vi "alinha-com-parede.vi"(4 "NXT/EV3":T1) -> (1 "NXT/EV3 2":T1)   [LabVIEW 2016]
uses:
  <vilib>/NXT/Subs/LVHSConnector.ctl
  <vilib>/NXT/LegoClasses/BrickReference/BrickReference.lvclass
  <vilib>/NXT/Block Support/NXT_InputPort.ctl
  <vilib>/NXT/Block Support/NXT_OutputPort.ctl
  <vilib>/NXT/Dual Mode Library/Sensors/Touch_Pressed.vi
  <vilib>/NXT/NXTIO Xnodes/NXTIONodeSubVIs/NXTMoveMotors.vi
  <vilib>/NXT/NXTIO Xnodes/AddressXNode/NXTIOAddress.xnode
  <vilib>/NXT/NXTIO Xnodes/NXTIOXNode/NXTIO.xnode
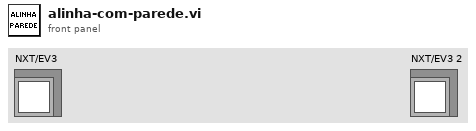
[diagram p1: front panel]
types:
  T1 = typedef "LVHSConnector.ctl" = refnum<class "BrickReference.lvclass">
  T2 = typedef "NXT_OutputPort.ctl" = u8
  T3 = typedef "NXT_InputPort.ctl" = u32
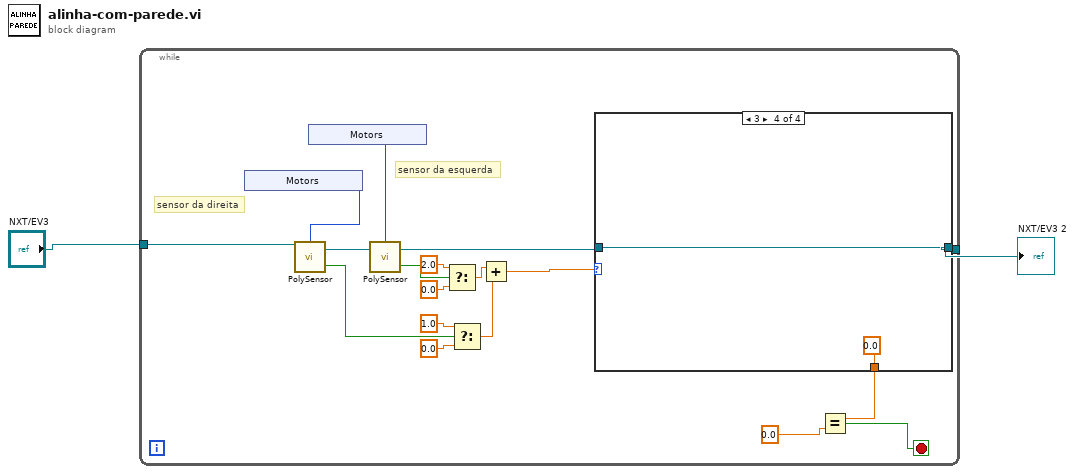
[diagram p0: block diagram]
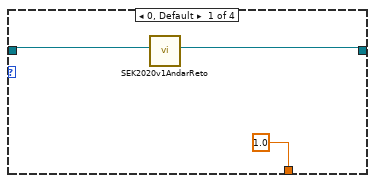
[diagram p2: hidden frame]
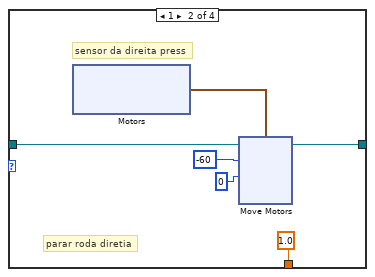
[diagram p3: hidden frame]
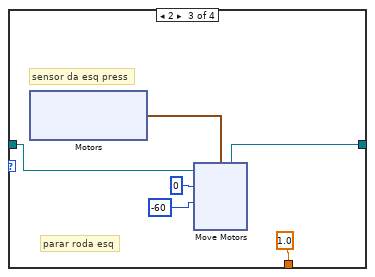
[diagram p4: hidden frame]
diagram:
  n1 = while {
    tunnel: "NXT/EV3" -> [w3]
    tunnel: [w13] -> w1
    stop <- w10 stop-if-true
    # "sensor da esquerda"
    # "sensor da direita"
    n2 = xnode "Motors"() -> ("Sensor"=w9:T3)
    n3 = call-poly <vilib>:"PolySensor.vi"("NXT/EV3"=w3, "Port (Port 1)"=w9) -> ("Yes / No"=w19:bool, "NXT/EV3"=w20:T1)  [unwired: 1 in]
    n4 = xnode "Motors"() -> ("Sensor"=w8:T3)
    n5 = call-poly <vilib>:"PolySensor.vi"("NXT/EV3"=w20, "Port (Port 1)"=w8) -> ("Yes / No"=w14:bool, "NXT/EV3"=w4:T1)  [unwired: 1 in]
    n6 = Select(t=2.0, s=w14, f=0.0 ("t")) -> (s? t:f=w7:dbl)
    n7 = Select(t=1.0, s=w19, f=0.0 ("t")) -> (s? t:f=w6:dbl)
    n8 = Add(x=w7, y=w6) -> (x+y=w5:dbl)
    n9 = case shown="3" w5 {
      tunnel: w4 -> [w24 w28 w43 w57]
      tunnel: [w25 w27 w42 w57] -> w13
      tunnel: [1.0 ("t") 1.0 ("t") 1.0 ("t") 0.0 ("t")] -> w12
      frame 0, Default {
        n10 = call "SEK2020v1AndarReto.vi"("NXT/EV3"=w24) -> ("NXT/EV3 2"=w25:T1)  [unwired: 9 in]
      }
      frame 1 {
        # "parar roda diretia"
        # "sensor da direita press"
        n11 = xnode "Motors"() -> ("Motor"=w29:cluster{"Port":T2, "Port":T2})
        n12 = xnode "Move Motors"("Power/Speed 1"=i8 -60, "Motors"=w29, "NXT/EV3"=w28, "Power/Speed 2"=i8 0) -> ("NXT/EV3"=w27:T1)
      }
      frame 2 {
        # "parar roda esq"
        # "sensor da esq press"
        n13 = xnode "Motors"() -> ("Motor"=w46:cluster{"Port":T2, "Port":T2})
        n14 = xnode "Move Motors"("Power/Speed 2"=i8 -60 ("Power/Speed 1"), "Power/Speed 1"=i8 0 ("Power/Speed 2"), "Motors"=w46, "NXT/EV3"=w43) -> ("NXT/EV3"=w42:T1)
      }
      frame 3 {
      }
    }
    n15 = Equal?(x=w12, y=0.0 ("t")) -> (x = y?=w10:bool)
  }
  "NXT/EV3 2" <- w1
